vi "p2.vi"() -> ()   [LabVIEW 2021, in "d6.lvlib"]
uses:
  d6.lvlib
  b9a53ecd-5d2b-482d-ade4-479f8d8c8092.vi
  AOC/AOC.lvlib
panel:
  in  "Example":string="nznrnfrfntjfmvfwmzdfjlvtqnbhcprsg"
  in  "Example":bool
  out "Answer":i64
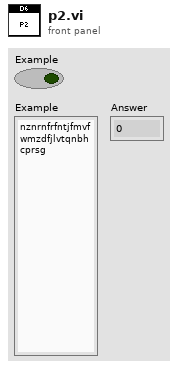
[diagram p1: front panel]
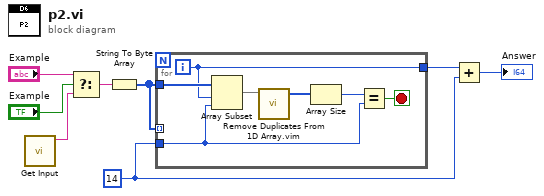
[diagram p0: block diagram]
diagram:
  w1 = 14 ("length")
  n1 = call "Get Input.vi"() -> ("Input"=w8:string)  [unwired: 11 in]
  n2 = Select(t="Example", s="Example", f=w8) -> (s? t:f=w3:string)
  n3 = String To Byte Array(string=w3) -> (unsigned byte array=w5:u8[])
  n4 = for {
    tunnel: w5 -> [_] mode=indexing
    tunnel: w5 -> [w15]
    tunnel: [w10] -> w4
    tunnel: w1 -> [w9]
    i -> [w10]
    stop <- w11 stop-if-true
    n5 = Array Subset(array=w15, index=w10, length=w9) -> (w14:u8[])
    n6 = call "Remove Duplicates From 1D Array.vim"("array"=w14) -> ("array with duplicates removed"=w13:u8[])  [unwired: 10 in]
    n7 = Array Size(array=w13) -> (size(s)=w12:i32)
    n8 = Equal?(x=w12, y=w9) -> (x = y?=w11:bool)
  }
  n9 = Add(x=w4, y=w1) -> (x+y=→"Answer":i32)
